vi "Add Class.vi"(8 "error in (no error)":errorcluster, 10 "Class":refnum<class>, 11 "Tag Tree In":refnum<class "LVCLass Tree.lvclass">) -> (0 "error out":errorcluster, 3 "Tag Tree Out":refnum<class "LVCLass Tree.lvclass">)   [LabVIEW 2020, in "Tree Helpers.lvlib" / "LVCLass Tree.lvclass"]
uses:
  LVCLass Tree.lvclass
  LVCLass Tree.lvclass/LVCLass Tree.ctl
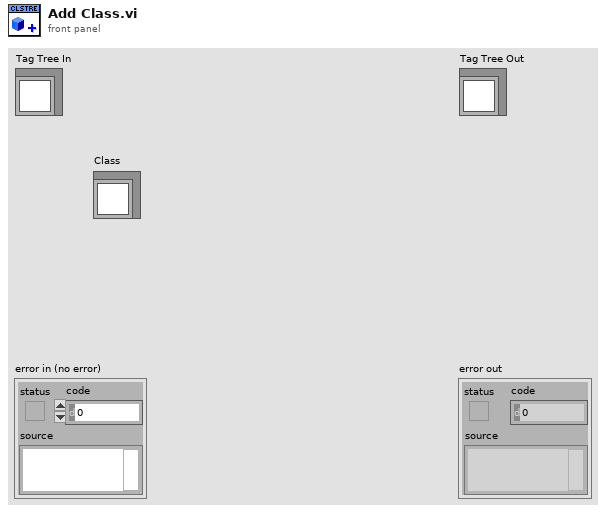
[diagram p1: front panel]
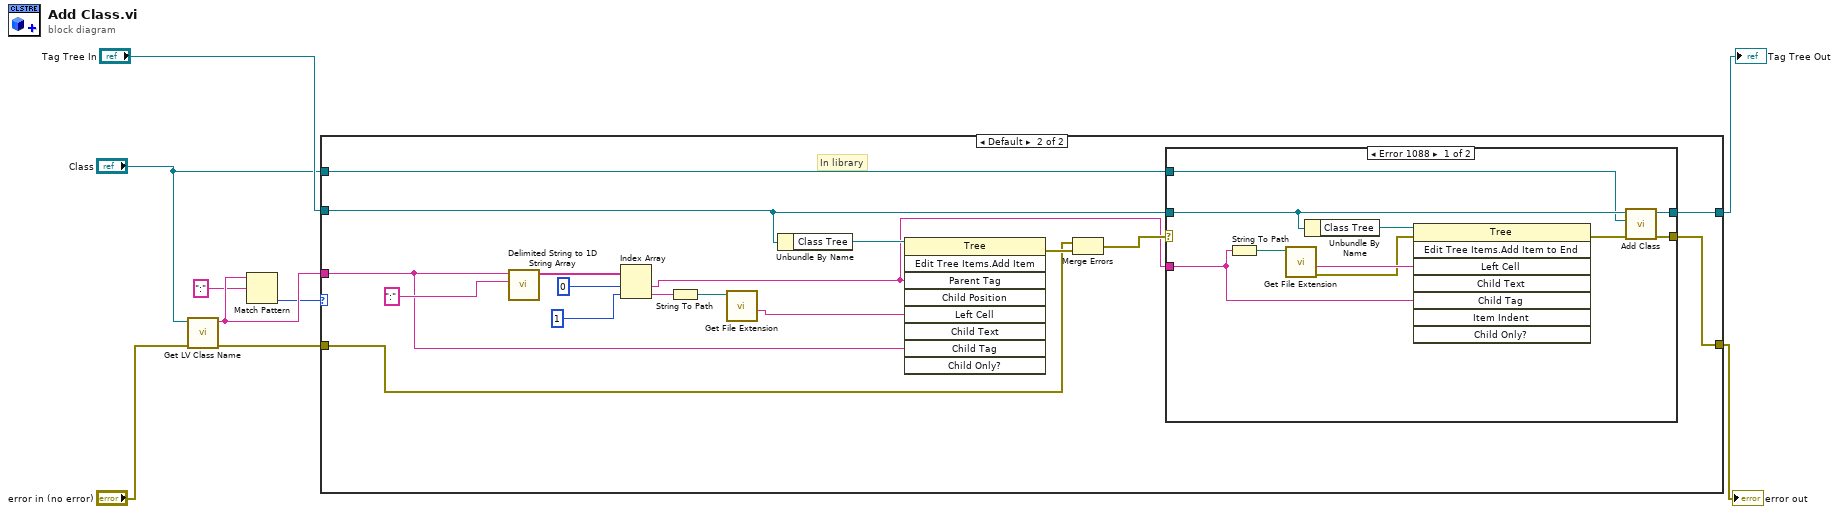
[diagram p0: block diagram]
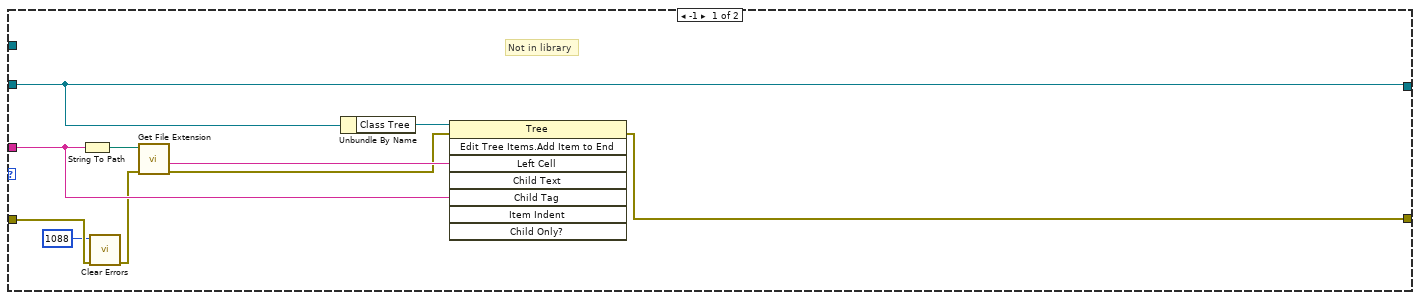
[diagram p2: hidden frame]
diagram:
  n1 = call <vilib>:"Get LV Class Name.vi"("error in (no error)"="error in (no error)", "object"="Class") -> ("error out"=w3:errorcluster, "class name"=w4:string)  [unwired: 8 in]
  n2 = Match Pattern(string=w4, regular expression=":") -> (offset past match=w2:i32)  [unwired: 1 in, 3 out]
  n3 = case shown="Default" w2 {
    tunnel: [w17 w33] -> w5
    tunnel: "Tag Tree In" -> [w18 w32]
    tunnel: [w18 w31] -> w6
    tunnel: w3 -> [w12 w27]
    tunnel: w4 -> [w13 w24]
    tunnel: "Class" -> [_ w20]
    frame -1 {
      # "Not in library"
      n4 = String To Path(string=w13) -> (path=w16:path)
      n5 = call <vilib>:"Clear Errors.vi"("error in (no error)"=w12, "specific error code to clear (0: all)"=1088) -> ("error out"=w10:errorcluster)  [unwired: 4 in, 1 out]
      n6 = call <vilib>:"Get File Extension.vi"("error in (no error)"=w10, "file"=w16) -> ("error out"=w14:errorcluster, "filename without extension"=w15:string)  [unwired: 5 in, 3 out]
      n7 = Unbundle By Name(w18) -> ("Class Tree"=w19:refnum<vi>)
      n8 = invoke on="Invoke Node" class="Tree" method="Edit Tree Items.Add Item to End"(reference=w19, error in=w14, "Left Cell"=w15, "Child Tag"=w13) -> (error out=w17:errorcluster)  [unwired: 4 in, 7 out]
    }
    frame Default {
      # "In library"
      n9 = call <vilib>:"Delimited String to 1D String Array.vi"("delimiter"=":", "delimited string"=w24) -> ("string array"=w30:string[])  [unwired: 9 in]
      n10 = Index Array(array=w30, index #1=0 ("index"), index #2=1 ("index")) -> (element #1=w21:string, element #2=w26:string)
      n11 = String To Path(string=w26) -> (path=w29:path)
      n12 = call <vilib>:"Get File Extension.vi"("file"=w29) -> ("filename without extension"=w25:string)  [unwired: 6 in, 4 out]
      n13 = Unbundle By Name(w32) -> ("Class Tree"=w36:refnum<vi>)
      n14 = invoke on="Invoke Node" class="Tree" method="Edit Tree Items.Add Item"(reference=w36, "Parent Tag"=w21, "Left Cell"=w25, "Child Tag"=w24) -> (error out=w34:errorcluster)  [unwired: 5 in, 8 out]
      n15 = Merge Errors(w27, w34) -> (w28:errorcluster)
      n16 = case shown="Error 1088" w28 {
        selector: w28 -> [_ w47]
        tunnel: [w38 w47] -> w33
        tunnel: w32 -> [w40 w48]
        tunnel: [w41 w48] -> w31
        tunnel: w21 -> [w44 _]
        tunnel: w20 -> [w37 _]
        frame #0 {
          n17 = String To Path(string=w44) -> (path=w45:path)
          n18 = call <vilib>:"Get File Extension.vi"("file"=w45) -> ("error out"=w42:errorcluster, "filename without extension"=w43:string)  [unwired: 6 in, 3 out]
          n19 = Unbundle By Name(w40) -> ("Class Tree"=w46:refnum<vi>)
          n20 = invoke on="Invoke Node" class="Tree" method="Edit Tree Items.Add Item to End"(reference=w46, error in=w42, "Left Cell"=w43, "Child Tag"=w44) -> (error out=w39:errorcluster)  [unwired: 4 in, 7 out]
          n21 = call "Add Class.vi"("error in (no error)"=w39, "Class"=w37, "Tag Tree In"=w40) -> ("error out"=w38:errorcluster, "Tag Tree Out"=w41:refnum<class "LVCLass Tree.lvclass">)  [unwired: 7 in]
        }
        frame #1 {
        }
      }
    }
  }
  "error out" <- w5
  "Tag Tree Out" <- w6
